vi "Start Acquisition.vi"(8 "error in (no error)":errorcluster, 11 "Process in":refnum<class "Process.lvclass">) -> (0 "error out":errorcluster, 3 "Process out":refnum<class "Process.lvclass">)   [LabVIEW 2025, in "Process Actor.lvlib" / "Process.lvclass"]
doc: "This method will cause the actor to sends its caller a stream of random numbers at a rate of 1 Hz."
uses:
  Process.lvclass
  Process.lvclass/Process.ctl
  Process Messages/Update Msg/Update Msg.lvclass
  <vilib>/ActorFramework/Actor/Actor.lvclass
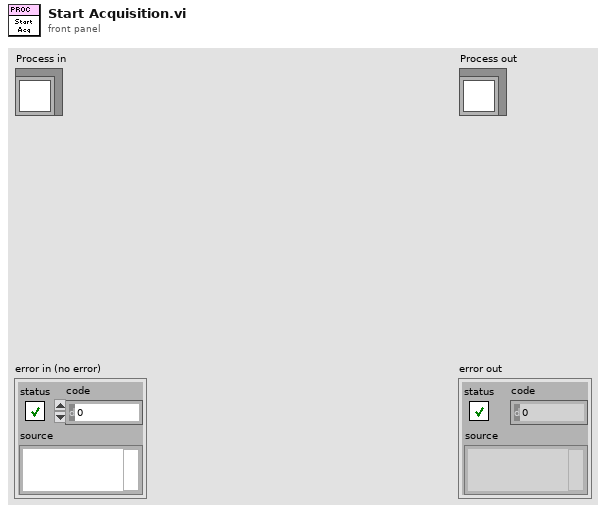
[diagram p1: front panel]
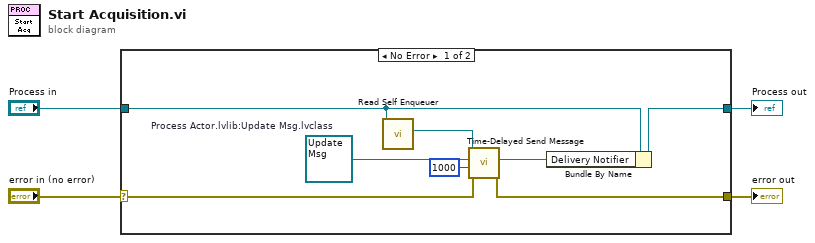
[diagram p0: block diagram]
diagram:
  n1 = case shown="No Error" "error in (no error)" {
    selector: "error in (no error)" -> [w9 w14]
    tunnel: [w8 w14] -> w3
    tunnel: [w6 w13] -> w1
    tunnel: "Process in" -> [w7 w13]
    frame No Error {
      w12 = refnum<class "Update Msg.lvclass"> refnum  # Process Actor.lvlib:Update Msg.lvclass
      n2 = call <vilib>:"Read Self Enqueuer.vi"("Actor"=w7) -> ("Self Enqueuer"=w11:refnum<class "Message Enqueuer.lvclass">)  [unwired: 10 in]
      n3 = call <vilib>:"Time-Delayed Send Message.vi"("error in (no error)"=w9, "Milliseconds To Wait"=1000, "Message"=w12, "Message Enqueuer"=w11) -> ("error out"=w8:errorcluster, "Delivery Notifier"=w5:refnum<notifier>)  [unwired: 6 in]
      n4 = Bundle By Name(cluster=w7, "Delivery Notifier"=w5) -> (w6:refnum<class "Process.lvclass">)
    }
    frame Error {
    }
  }
  "error out" <- w3
  "Process out" <- w1
